vi "Get Dependency.vi"(8 "error in (no error)":errorcluster, 11 "LogEngine":refnum<class "LogEngine.lvclass">) -> (0 "error out":errorcluster, 2 "Dependency":T1, 3 "LogEngine out":refnum<class "LogEngine.lvclass">)   [LabVIEW 2022 SP3, in "LogEngine.lvclass"]
doc: "Developed by Kevin Thompson\nkevin@thompsonengineering.net\n\nCopyright 2018-2020\nThompson Engineering, LLC"
uses:
  LogEngine.lvclass
  LogEngine.lvclass/LogEngine.ctl
  Support/DataQueues/DataQueues.lvclass
  DAQ/DAQ.lvclass
  Data Types/Dependency--cluster.ctl
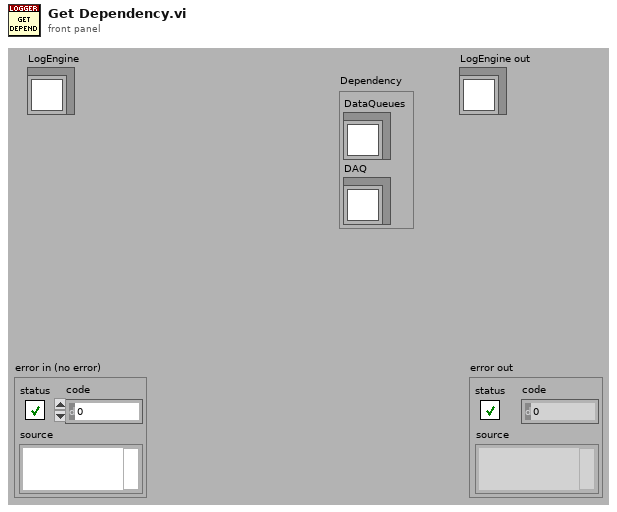
[diagram p1: front panel]
types:
  T1 = typedef "LogEngine.lvclass/Dependency--cluster.ctl" = cluster{"DataQueues":refnum<class "DataQueues.lvclass">, "DAQ":refnum<class "DAQ.lvclass">}
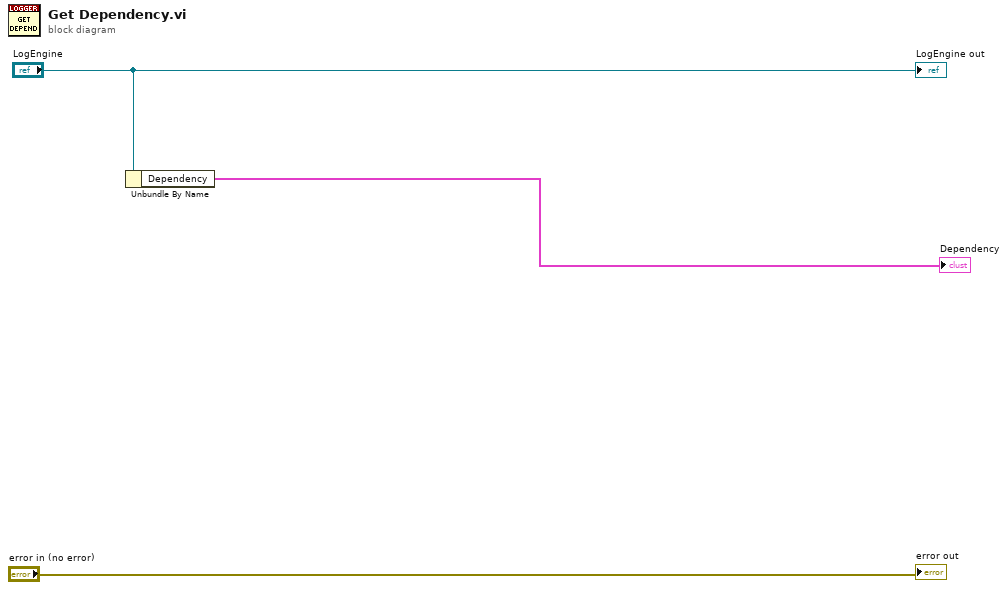
[diagram p0: block diagram]
diagram:
  n1 = Unbundle By Name("LogEngine") -> ("Dependency"=→"Dependency":T1)
  "error out" <- "error in (no error)"
  "LogEngine out" <- "LogEngine"
